vi "Output Lines.vi"(7 "error in (no error)":errorcluster, 8 "position (0, 0)":cluster{"row":i8, "column":i8}, 9 "character codes":u8[](array[numeric]), 10 "cluster of private data in":T1={"FPGA VI Reference"=refnum, "device index"=0, "screen size"=enum."8x1", "font size"=enum."5x8", "auto wrap"=FALSE, "alignment"=enum."None", "number of line"=enum."2 lines", "shift 0"=0, "entry mode 0"=enum."increment & no shift", "shift 1"=0, "entry mode 1"=enum."increment & no shift"}) -> (0 "error out":errorcluster, 1 "current position":cluster{"row":i8, "column":i8}, 3 "cluster of private data out":T1={"FPGA VI Reference"=refnum, "device index"=0, "screen size"=enum."8x1", "font size"=enum."5x8", "auto wrap"=FALSE, "alignment"=enum."None", "number of line"=enum."2 lines", "shift 0"=0, "entry mode 0"=enum."increment & no shift", "shift 1"=0, "entry mode 1"=enum."increment & no shift"})   [LabVIEW 2017, in "HD44780.lvclass"]
uses:
  HD44780.lvclass
  Common/HD44780 Common.lvlib
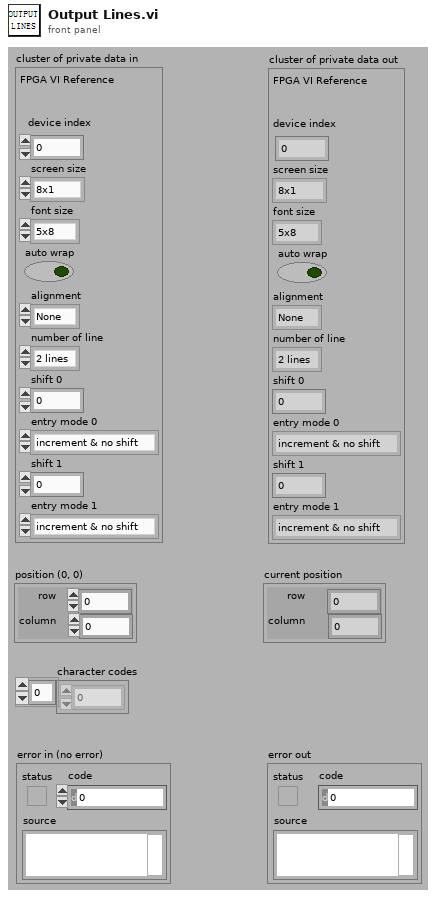
[diagram p1: front panel]
types:
  T1 = cluster{"FPGA VI Reference":refnum<k20>, "device index":i8, "screen size":enum8{"8x1", "8x2", "12x4", "16x1", "16x2", "16x4", "20x1", "20x2", "20x4", "24x1", "24x2", "40x2", "40x4"}, "font size":enum8{"5x8", "5x10"}, "auto wrap":bool, "alignment":enum16{"None", "Left", "Center", "Right"}, "number of line":enum8{"1 line", "2 lines"}, "shift 0":i8, "entry mode 0":enum8{"increment & no shift", "increment & shift", "decrement & no shift", "decrement & shift"}, "shift 1":i8, "entry mode 1":enum8{"increment & no shift", "increment & shift", "decrement & no shift", "decrement & shift"}}
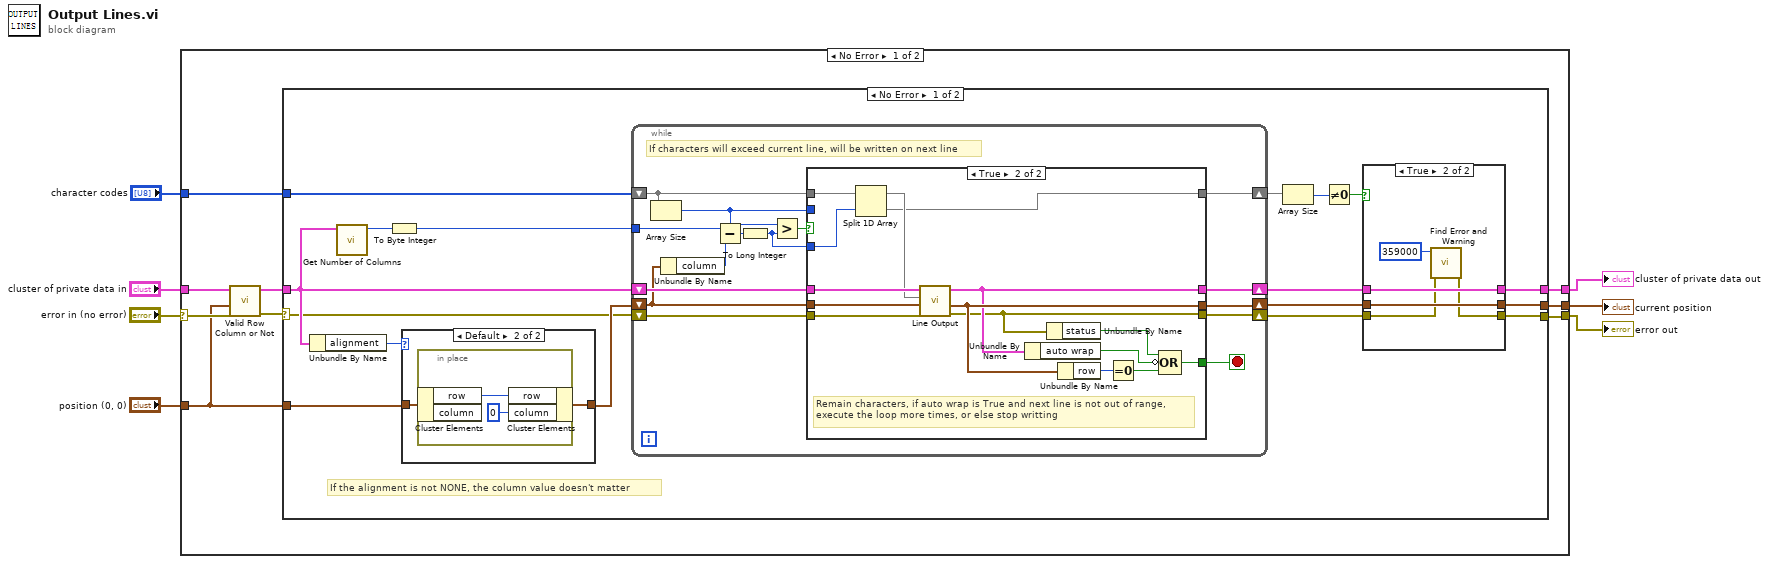
[diagram p0: block diagram]
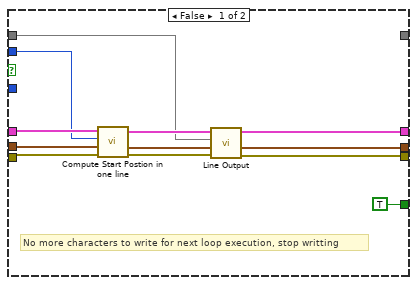
[diagram p4: hidden frame]
diagram:
  n1 = case shown="No Error" "error in (no error)" {
    selector: "error in (no error)" -> [w10 w94]
    tunnel: [w13 w94] -> w7
    tunnel: "position (0, 0)" -> [w8 w92]
    tunnel: "character codes" -> [w16 _]
    tunnel: [w14 w92] -> w4
    tunnel: [w15 w93] -> w1
    tunnel: "cluster of private data in" -> [w12 w93]
    frame No Error {
      n2 = call "Valid Row Column or Not.vi"("error in (no error)"=w10, "cursor position in"=w8, "cluster of private data in"=w12) -> ("error out"=w9:errorcluster, "cluster of private data out"=w11:T1)  [unwired: 6 in, 1 out]
      n3 = case shown="No Error" w9 {
        selector: w9 -> [w27 w91]
        tunnel: w16 -> [w33 _]
        tunnel: [w21 w90] -> w15
        tunnel: [w19 w89] -> w14
        tunnel: [w17 w91] -> w13
        tunnel: w11 -> [w28 w90]
        tunnel: w8 -> [w26 w89]
        frame No Error {
          # "If the alignment is not NONE, the column value doesn't matter"
          n4 = Unbundle By Name(w28) -> ("alignment"=w31:enum16{"None", "Left", "Center", "Right"})
          n5 = call "Get Number of Columns.vi"("cluster of private data in"=w28) -> ("column number"=w32:u8)  [unwired: 10 in]
          n6 = To Byte Integer(number=w32) -> (8bit integer=w29:i8)
          n7 = case shown="Default" w31 {
            tunnel: w26 -> [w42 w44]
            tunnel: [w42 w43] -> w30
            frame "None" {
            }
            frame Default {
              n8 = in-place {
                n9 = in-place-cluster #1(w44) -> ("row"=w46:i8)  [unwired: 1 out]
                n10 = in-place-cluster #1("row"=w46, "column"=i8 0) -> (w43:cluster{"row":i8, "column":i8})
              }
            }
          }
          n11 = while {
            shift-right: [w57] -> w25
            shift-left: w33 -> [w58]
            tunnel: w29 -> [w48]
            shift-right: [w55] -> w20
            shift-left: w30 -> [w51]
            shift-right: [w53] -> w22
            shift-left: w28 -> [w60]
            shift-right: [w52] -> w18
            shift-left: w27 -> [w59]
            stop <- w54 stop-if-true
            # "If characters will exceed current line, will be written on next line"
            n12 = Array Size(array=w58) -> (size(s)=w56:i32)
            n13 = Unbundle By Name(w51) -> ("column"=w50:i8)
            n14 = Subtract(x=w48, y=w50) -> (x-y=w49:i8)
            n15 = To Long Integer(number=w49) -> (32bit integer=w47:i32)
            n16 = Greater?(x=w56, y=w47) -> (0:w61:bool)
            n17 = case shown="True" w61 {
              tunnel: w60 -> [w73 w88]
              tunnel: w59 -> [w72 w87]
              tunnel: w51 -> [w70 w86]
              tunnel: w58 -> [w67 w85]
              tunnel: w47 -> [_ w84]
              tunnel: [_ w82] -> w57
              tunnel: w56 -> [w71 _]
              tunnel: [w65 w79] -> w53
              tunnel: [w64 w75] -> w52
              tunnel: [w63 w80] -> w55
              tunnel: [TRUE w76] -> w54
              frame False {
                # "No more characters to write for next loop execution, stop writting"
                n18 = call "Compute Start Postion in one line.vi"("error in (no error)"=w72, "original position"=w70, "string length in"=w71, "cluster of private data in"=w73) -> ("error out"=w69:errorcluster, "output position"=w66:cluster{"row":i8, "column":i8}, "cluster of private data out"=w68:T1)  [unwired: 3 in, 1 out]
                n19 = call "Line Output.vi"("error in (no error)"=w69, "position (0, 0)"=w66, "character codes"=w67, "cluster of private data in"=w68) -> ("error out"=w64:errorcluster, "current position"=w63:cluster{"row":i8, "column":i8}, "cluster of private data out"=w65:T1)  [unwired: 5 in]
              }
              frame True {
                # "Remain characters, if auto wrap is True and next line is not out of range,\nexecute the loop more times, or else stop writting"
                n20 = Split 1D Array(array=w85, index=w84) -> (first subarray=w83:u8[], second subarray=w82:u8[])
                n21 = call "Line Output.vi"("error in (no error)"=w87, "position (0, 0)"=w86, "character codes"=w83, "cluster of private data in"=w88) -> ("error out"=w75:errorcluster, "current position"=w80:cluster{"row":i8, "column":i8}, "cluster of private data out"=w79:T1)  [unwired: 5 in]
                n22 = Unbundle By Name(w79) -> ("auto wrap"=w77:bool)
                n23 = Unbundle By Name(w75) -> ("status"=w74:bool)
                n24 = Unbundle By Name(w80) -> ("row"=w81:i8)
                n25 = Equal To 0?(x=w81) -> (x = 0?=w78:bool)
                n26 = Compound Arithmetic op=OR(w74, invert w77, w78) -> (w76:bool)
              }
            }
          }
          n27 = Array Size(array=w25) -> (size(s)=w24:i32)
          n28 = Not Equal To 0?(x=w24) -> (x != 0?=w23:bool)
          n29 = case shown="True" w23 {
            tunnel: w22 -> [w36 w41]
            tunnel: [w36 w41] -> w21
            tunnel: w20 -> [w35 w40]
            tunnel: [w35 w40] -> w19
            tunnel: w18 -> [w34 w38]
            tunnel: [w34 w37] -> w17
            frame False {
            }
            frame True {
              n30 = call "Find Error and Warning.vi"("error in (no error)"=w38, "error code"=359000) -> ("error out"=w37:errorcluster)  [unwired: 9 in]
            }
          }
        }
        frame Error {
        }
      }
    }
    frame Error {
    }
  }
  "error out" <- w7
  "current position" <- w4
  "cluster of private data out" <- w1
